vi "TrapBlankChan.vi"(11 "error in (no error)":errorcluster) -> (1 "message":string, 3 "error out":errorcluster)   [LabVIEW 2010]
uses:
  <vilib>/Utility/error.llb/DialogType.ctl
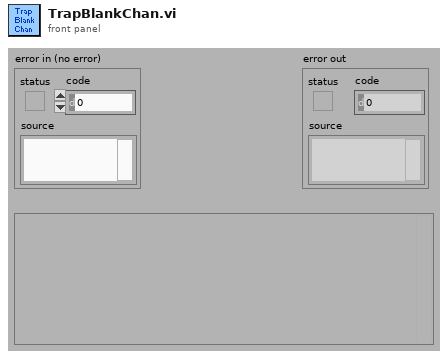
[diagram p1: front panel]
types:
  T1 = typedef "DialogType.ctl" = u16
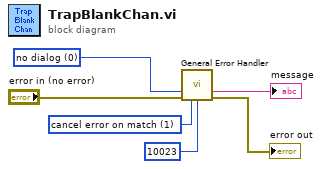
[diagram p0: block diagram]
diagram:
  w4 = T1 0 items=["no dialog", "OK message", "continue or stop message", "OK message + warnings", "continue/stop + warnings"] ("type of dialog (OK msg:1)")
  w6 = 1 items=["no exception", "cancel error on match", "set error on match"] ("[exception action] (none:0)")
  n1 = call <vilib>:"General Error Handler.vi"("type of dialog (OK msg:1)"=w4, "error in (no error)"="error in (no error)", "[exception action] (none:0)"=w6, "[exception code]"=10023) -> ("message"=→"message":string, "error out"=→"error out":errorcluster)  [unwired: 7 in, 3 out]
